vi "plot_splitYoung.vi"(9 "Input Arrays":dbl[][](array[numeric])=[[1.0, 4.0, 7.0], [2.0, 5.0, 8.0], [3.0, 6.0, 9.0]]) -> (10 "output cluster":T1)   [LabVIEW 2018]
doc: "Adds the datapoints for Timestamp, Rain Rate, and Accumulation to their corresponding plot arrays."
panel:
  out "Young Wind Speed":dbl[](array[numeric])
  out "Young Pressure":dbl[](array[numeric])
  out "Young Humidity":dbl[](array[numeric])
  out "Young Rain Fall":dbl[](array[numeric])
  out "Young Rain Rate":dbl[](array[numeric])
  out "Young Wind Direction":dbl[](array[numeric])
  out "Young Temperature":dbl[](array[numeric])
  out "Timestamp":dbl[](array[numeric])
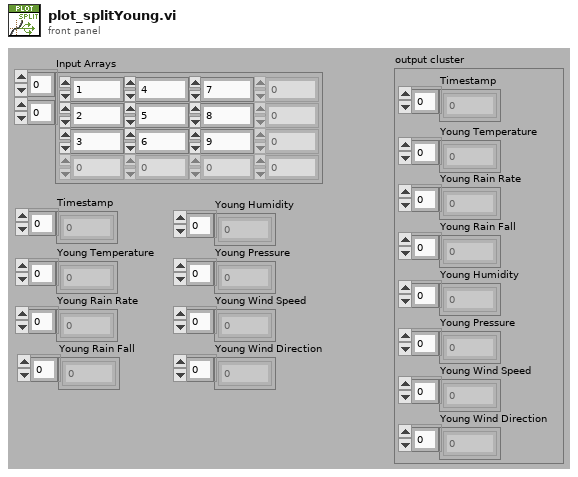
[diagram p1: front panel]
types:
  T1 = cluster{"Timestamp":dbl[], "Young Temperature":dbl[], "Young Rain Rate":dbl[], "Young Rain Fall":dbl[], "Young Humidity":dbl[], "Young Pressure":dbl[], "Young Wind Speed":dbl[], "Young Wind Direction":dbl[]}
  T2 = cluster{"Input Arrays":dbl[], "Input Arrays":dbl[], "Input Arrays":dbl[], "Input Arrays":dbl[], "Input Arrays":dbl[], "Input Arrays":dbl[], "Input Arrays":dbl[], "Input Arrays":dbl[]}
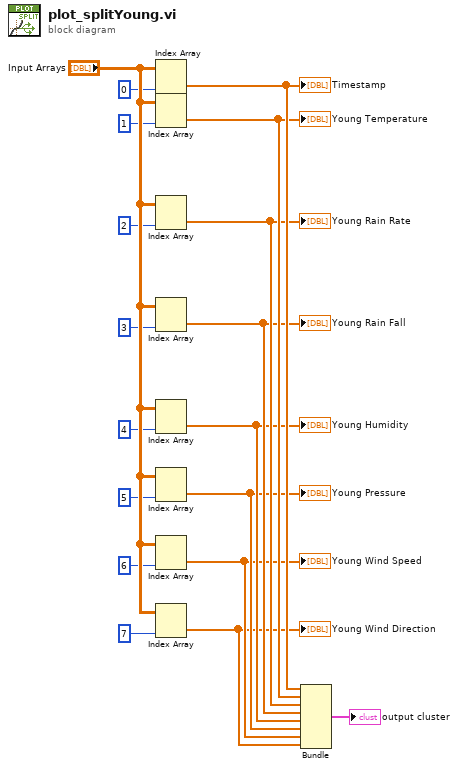
[diagram p0: block diagram]
diagram:
  n1 = Index Array(array="Input Arrays", index (col)=0 ("disabled index (col)")) -> (element=w9:dbl[])  [unwired: 1 in]
  "Timestamp" <- w9
  n2 = Index Array(array="Input Arrays", index (col)=1 ("disabled index (col)")) -> (element=w8:dbl[])  [unwired: 1 in]
  "Young Temperature" <- w8
  n3 = Index Array(array="Input Arrays", index (col)=2 ("disabled index (col)")) -> (element=w7:dbl[])  [unwired: 1 in]
  "Young Rain Rate" <- w7
  n4 = Index Array(array="Input Arrays", index (col)=3 ("disabled index (col)")) -> (element=w6:dbl[])  [unwired: 1 in]
  "Young Rain Fall" <- w6
  n5 = Index Array(array="Input Arrays", index (col)=4 ("disabled index (col)")) -> (element=w5:dbl[])  [unwired: 1 in]
  "Young Humidity" <- w5
  n6 = Index Array(array="Input Arrays", index (col)=5 ("disabled index (col)")) -> (element=w4:dbl[])  [unwired: 1 in]
  "Young Pressure" <- w4
  n7 = Index Array(array="Input Arrays", index (col)=6 ("disabled index (col)")) -> (element=w3:dbl[])  [unwired: 1 in]
  "Young Wind Speed" <- w3
  n8 = Index Array(array="Input Arrays", index (col)=7 ("disabled index (col)")) -> (element=w2:dbl[])  [unwired: 1 in]
  "Young Wind Direction" <- w2
  n9 = Bundle("Input Arrays"=w9, "Input Arrays"=w8, "Input Arrays"=w7, "Input Arrays"=w6, "Input Arrays"=w5, "Input Arrays"=w4, "Input Arrays"=w3, "Input Arrays"=w2) -> (→"output cluster":T2)  [unwired: 1 in]
